vi "TcA06-003_ConstructorErrorHandling.vi"(1 "Input buffer":T3="1", 3 "Invocation info":T2, 5 "error in (no error)":errorcluster, 6 "Add log to result?":bool) -> (16 "Test Data":T1 {"Numeric Measurement" format="%.2f"}, 19 "error out":errorcluster)   [LabVIEW 2020]
doc: "Test case template."
uses:
  Shared/Support_InputBuffer.ctl
  Shared/Support_InvocationInfo.ctl
  Shared/Support_TestData.ctl
  TestClasses/G#SubSubClass1_class/G#SubSubClass1.lvclass
  C:/Projects/GsharpGIT/Verification/TestCases/TestClasses/G#BaseClass1_class/G#BaseClass1.lvclass
  TestClasses/G#BaseClass1_class/G#BaseClass1.lvclass
  <vilib>/addons/_AddQ/G#Object/G#Object.lvclass
panel:
  in  "Test name":string="TcA06-003 Constructor error handling"
  out "Test result":bool
  out "Result":string
  # "Verify that if a constructor is not used correct, an error will\nbe generated."
  # "Sub test case"
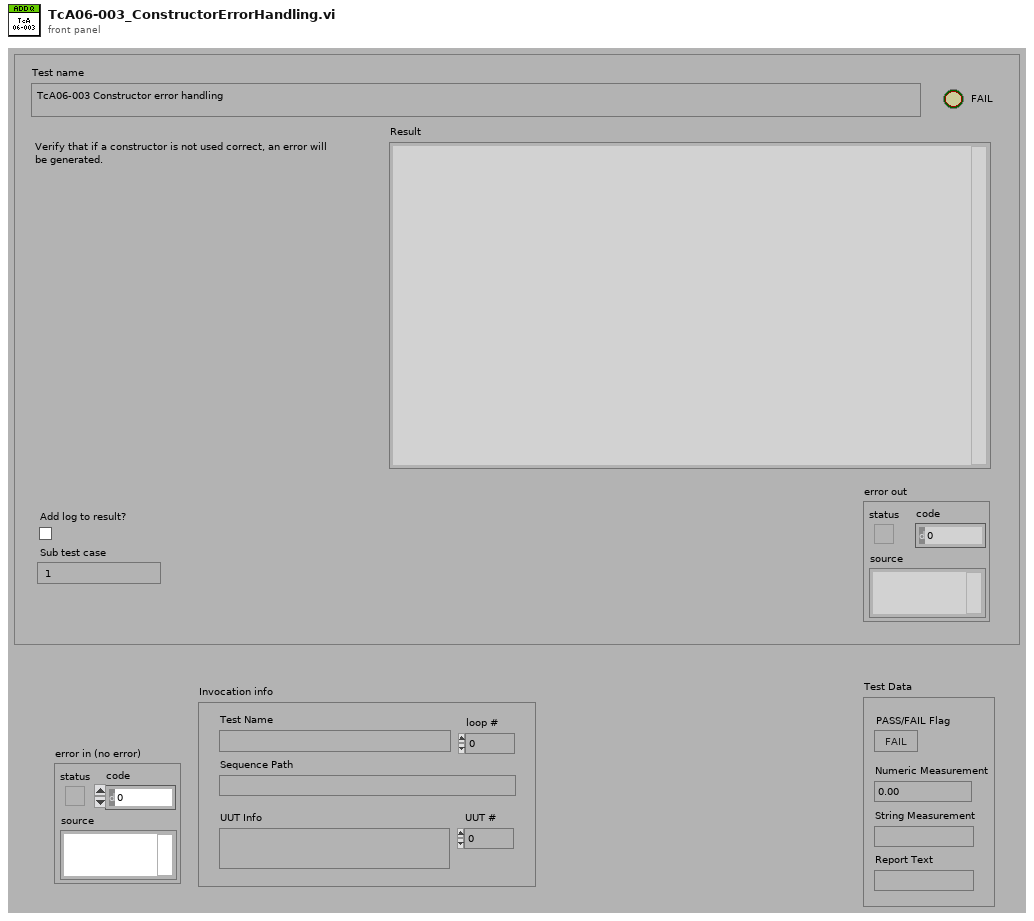
[diagram p1: front panel]
types:
  T1 = typedef "Support_TestData.ctl" = cluster{"PASS/FAIL Flag":bool, "Numeric Measurement":dbl, "String Measurement":string, "Report Text":string}
  T2 = typedef "Support_InvocationInfo.ctl" = cluster{"UUT #":i32, "loop #":i32, "UUT Info":string, "Test Name":string, "Sequence Path":path}
  T3 = typedef "Support_InputBuffer.ctl" = string
  T4 = typedef "Support_ResultType.ctl" = cluster{"Pass":bool, "Comment":string, "MeasurementValue":dbl}
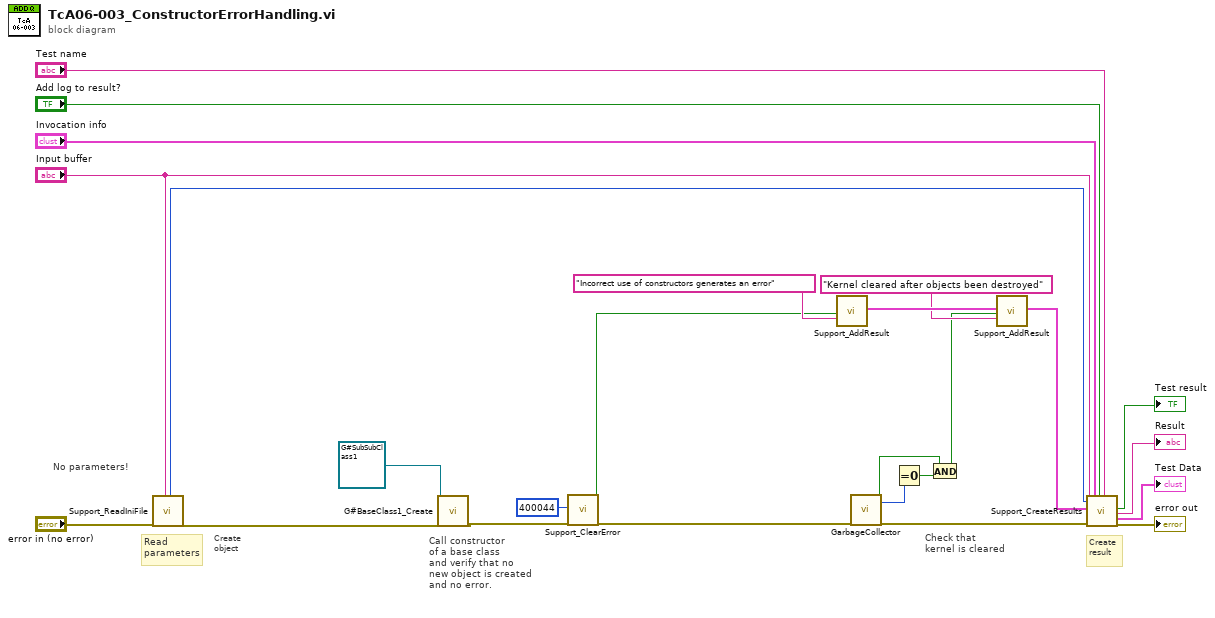
[diagram p0: block diagram]
diagram:
  # "Check that\nkernel is cleared"
  # "Call constructor\nof a base class\nand verify that no\nnew object is created\nand no error."
  # "No parameters!"
  # "Create\nobject"
  # "Create\nresult"
  # "Read\nparameters"
  n1 = call "Support_ReadIniFile.vi"("error in (no error)"="error in (no error)", "Sub test case"="Input buffer") -> ("Timer start"=w16:u32, "error out"=w10:errorcluster)  [unwired: 10 in, 6 out]
  n2 = call "G#BaseClass1_Create.vi"("reference in"=refnum<class "G#SubSubClass1.lvclass"> refnum ("G#SubSubClass1.lvclass"), "error in (no error)"=w10) -> ("error out"=w4:errorcluster)  [unwired: 15 in, 2 out]
  n3 = call "Support_ClearError.vi"("code"=400044, "error in (no error)"=w4) -> ("Cleared?"=w2:bool, "error out"=w3:errorcluster)  [unwired: 16 in]
  n4 = call "Support_AddResult.vi"("Pass"=w2, "Comment"="Incorrect use of constructors generates an error") -> ("Results out"=w13:T4[])  [unwired: 17 in]
  n5 = call <vilib>:"GarbageCollector.vi"("error in (no error)"=w3) -> ("OK"=w6:bool, "# of objects killed"=w8:i32, "error out"=w15:errorcluster)  [unwired: 16 in]
  n6 = Equal To 0?(x=w8) -> (x = 0?=w7:bool)
  n7 = And(x=w6, y=w7) -> (x .and. y?=w5:bool)
  n8 = call "Support_AddResult.vi"("Results in"=w13, "Pass"=w5, "Comment"="Kernel cleared after objects been destroyed") -> ("Results out"=w12:T4[])  [unwired: 16 in]
  n9 = call "Support_CreateResults.vi"("Sub test case"="Input buffer", "Timer start"=w16, "Results"=w12, "error in (no error)"=w15, "Invocation info"="Invocation info", "Add log to result?"="Add log to result?", "Test name"="Test name") -> ("Pass/fail flag"=→"Test result":bool, "Result"=→"Result":string, "Test Data"=→"Test Data":T1, "error out"=→"error out":errorcluster)  [unwired: 9 in]
